vi "Timer Initialize.vi"() -> (14 "Fatal Error Out":T11, 15 "State Out":T1)   [LabVIEW 2021, in "myRIO Create Timer IRQ.xnode"]
uses:
  <vilib>/myRIO/Instrument Drivers/IRQ/Timer IRQ/vis/myRIO Create Timer IRQ.xnode
  <vilib>/XNodeSupport/XNodeErrorCluster.ctl
  <vilib>/myRIO/Instrument Drivers/IRQ/Timer IRQ/vis/Timer State.ctl
  <vilib>/myRIO/Common/Instrument Driver Framework/Utilities/typedefs/myRIOXPeripheral.ctl
  <vilib>/XNodeSupport/XNodeTerm4Array.ctl
  <vilib>/XNodeSupport/XNodeTerm4.ctl
  <vilib>/XNodeSupport/XNodeString.ctl
  <vilib>/XNodeSupport/XNodeVariant.ctl
  <vilib>/XNodeSupport/XNodeRect32.ctl
  <vilib>/XNodeSupport/XNodeInt.ctl
  <vilib>/XNodeSupport/XNodeBool.ctl
  <vilib>/XNodeSupport/XNodeTermDirection.ctl
  <vilib>/myRIO/Common/Instrument Driver Framework/myRIO v1.0/IRQ/typedefs/Callback VI Ref.ctl
  <vilib>/myRIO/Common/Instrument Driver Framework/Utilities/vis/myRIOXGlobal.vi
  <vilib>/XNodeSupport/NI_XNodeSupport.lvlib
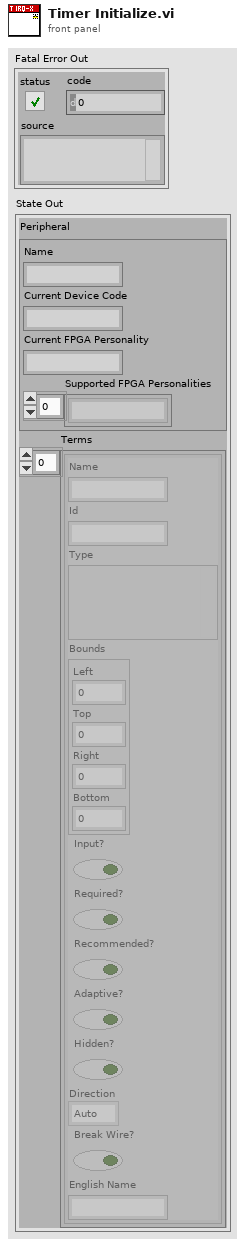
[diagram p1: front panel]
types:
  T1 = typedef "myRIO Create Timer IRQ.xnode/Timer State.ctl" = cluster{"Peripheral":T2, "Terms":T3}
  T2 = typedef "myRIOXPeripheral.ctl" = cluster{"Name":string, "Current Device Code":string, "Current FPGA Personality":string, "Supported FPGA Personalities":string[]}
  T3 = typedef "NI_XNodeSupport.lvlib/XNodeTerm4Array.ctl" = T4[]
  T4 = typedef "NI_XNodeSupport.lvlib/XNodeTerm4.ctl" = cluster{"Name":T5, "Id":T5, "Type":T6, "Bounds":T7, "Input?":T9, "Required?":T9, "Recommended?":T9, "Adaptive?":T9, "Hidden?":T9, "Direction":T10, "Break Wire?":T9, "English Name":T5}
  T5 = typedef "NI_XNodeSupport.lvlib/XNodeString.ctl" = string
  T6 = typedef "NI_XNodeSupport.lvlib/XNodeVariant.ctl" = variant
  T7 = typedef "NI_XNodeSupport.lvlib/XNodeRect32.ctl" = cluster{"Left":T8, "Top":T8, "Right":T8, "Bottom":T8}
  T8 = typedef "NI_XNodeSupport.lvlib/XNodeInt.ctl" = i32
  T9 = typedef "NI_XNodeSupport.lvlib/XNodeBool.ctl" = bool
  T10 = typedef "NI_XNodeSupport.lvlib/XNodeTermDirection.ctl" = enum32{"Auto", "Up", "Down", "Left", "Right", "Center"}
  T11 = typedef "NI_XNodeSupport.lvlib/XNodeErrorCluster.ctl" = errorcluster
  T12 = typedef "Callback VI Ref.ctl" = refnum<vi>
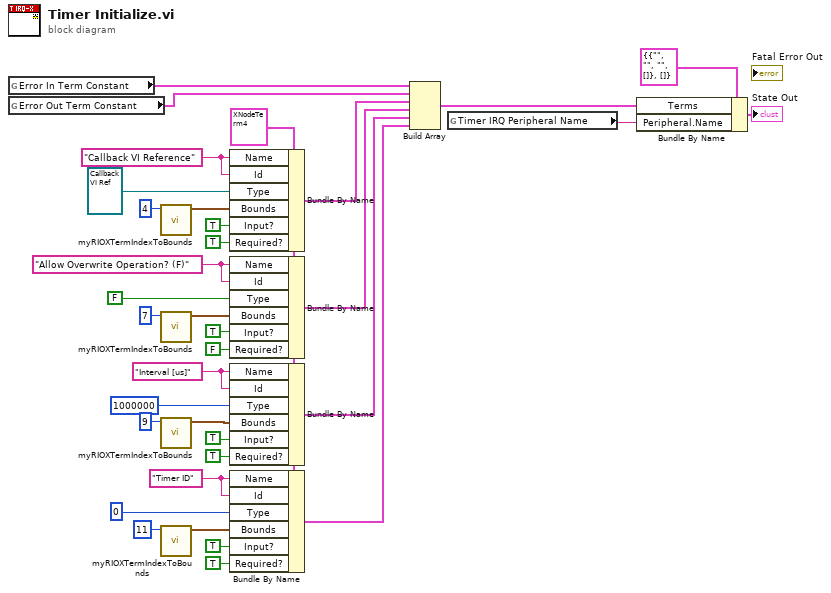
[diagram p0: block diagram]
diagram:
  w8 = T5 "Timer ID" ("Name")
  w13 = T5 "Interval [us]" ("Name")
  w20 = T5 "Allow Overwrite Operation? (F)" ("Name")
  w27 = T5 "Callback VI Reference" ("Name")
  w22 = T4 {"Name"="", "Id"="", "Type"=variant, "Bounds"={"Left"=0, "Top"=0, "Right"=0, "Bottom"=0}, "Input?"=FALSE, "Required?"=FALSE, "Recommended?"=FALSE, "Adaptive?"=FALSE, "Hidden?"=FALSE, "Direction"=enum."Auto", "Break Wire?"=FALSE, "English Name"=""} ("Error In Term Constant")
  n1 = global read "myRIOXGlobal.vi" "Error In Term Constant"() -> (w32:T4)
  n2 = global read "myRIOXGlobal.vi" "Error Out Term Constant"() -> (w31:T4)
  n3 = call <vilib>:"myRIOXTermIndexToBounds.vi"("Index"=4) -> ("Bounds"=w30:T7)  [unwired: 10 in]
  n4 = call <vilib>:"myRIOXTermIndexToBounds.vi"("Index"=7) -> ("Bounds"=w17:T7)  [unwired: 10 in]
  n5 = call <vilib>:"myRIOXTermIndexToBounds.vi"("Index"=9) -> ("Bounds"=w12:T7)  [unwired: 10 in]
  n6 = call <vilib>:"myRIOXTermIndexToBounds.vi"("Index"=11) -> ("Bounds"=w9:T7)  [unwired: 10 in]
  n7 = Bundle By Name(cluster=w22, "Name"=w27, "Id"=w27, "Type"=T12 refnum ("Callback VI"), "Bounds"=w30, "Input?"=T9 TRUE, "Required?"=T9 TRUE) -> (w25:T4)
  n8 = Bundle By Name(cluster=w22, "Name"=w20, "Id"=w20, "Type"=FALSE ("Allow Overwrite? (F)"), "Bounds"=w17, "Input?"=T9 TRUE, "Required?"=T9 FALSE) -> (w24:T4)
  n9 = Bundle By Name(cluster=w22, "Name"=w13, "Id"=w13, "Type"=u32 1000000 ("Interval(us)"), "Bounds"=w12, "Input?"=T9 TRUE, "Required?"=T9 TRUE) -> (w23:T4)
  n10 = Bundle By Name(cluster=w22, "Name"=w8, "Id"=w8, "Type"=u8 0 ("IRQ Number"), "Bounds"=w9, "Input?"=T9 TRUE, "Required?"=T9 TRUE) -> (w21:T4)
  n11 = Build Array(w32, w31, w25, w24, w23, w21) -> (w1:T4[])
  n12 = global read "myRIOXGlobal.vi" "Timer IRQ Peripheral Name"() -> (w33:string)
  n13 = Bundle By Name(cluster=T1 {"Peripheral"={"Name"="", "Current Device Code"="", "Current FPGA Personality"="", "Supported FPGA Personalities"=[]}, "Terms"=[]} ("State Out"), "Terms"=w1, "Peripheral.Name"=w33) -> (→"State Out":T1)
